vi "TextDiff.vi"(8 "error in (no error)":errorcluster, 9 "Output Folders":T5, 10 "VI 2 Screenshots in":T1, 11 "VI 1 Screenshots in":T1) -> (0 "error out":errorcluster, 2 "Description":string, 3 "appended path":path)   [LabVIEW 2020, in "VIDiffScreenshots.lvlib"]
uses:
  VIDiffScreenshots.lvlib
  Utilities/Output Folders.ctl
  VIScreenshots.ctl
  ScreenshotInfo.ctl
  Screenshot Type.ctl
  Utilities/FilePaths.ctl
  Utilities/VIDiffUtilities.lvlib
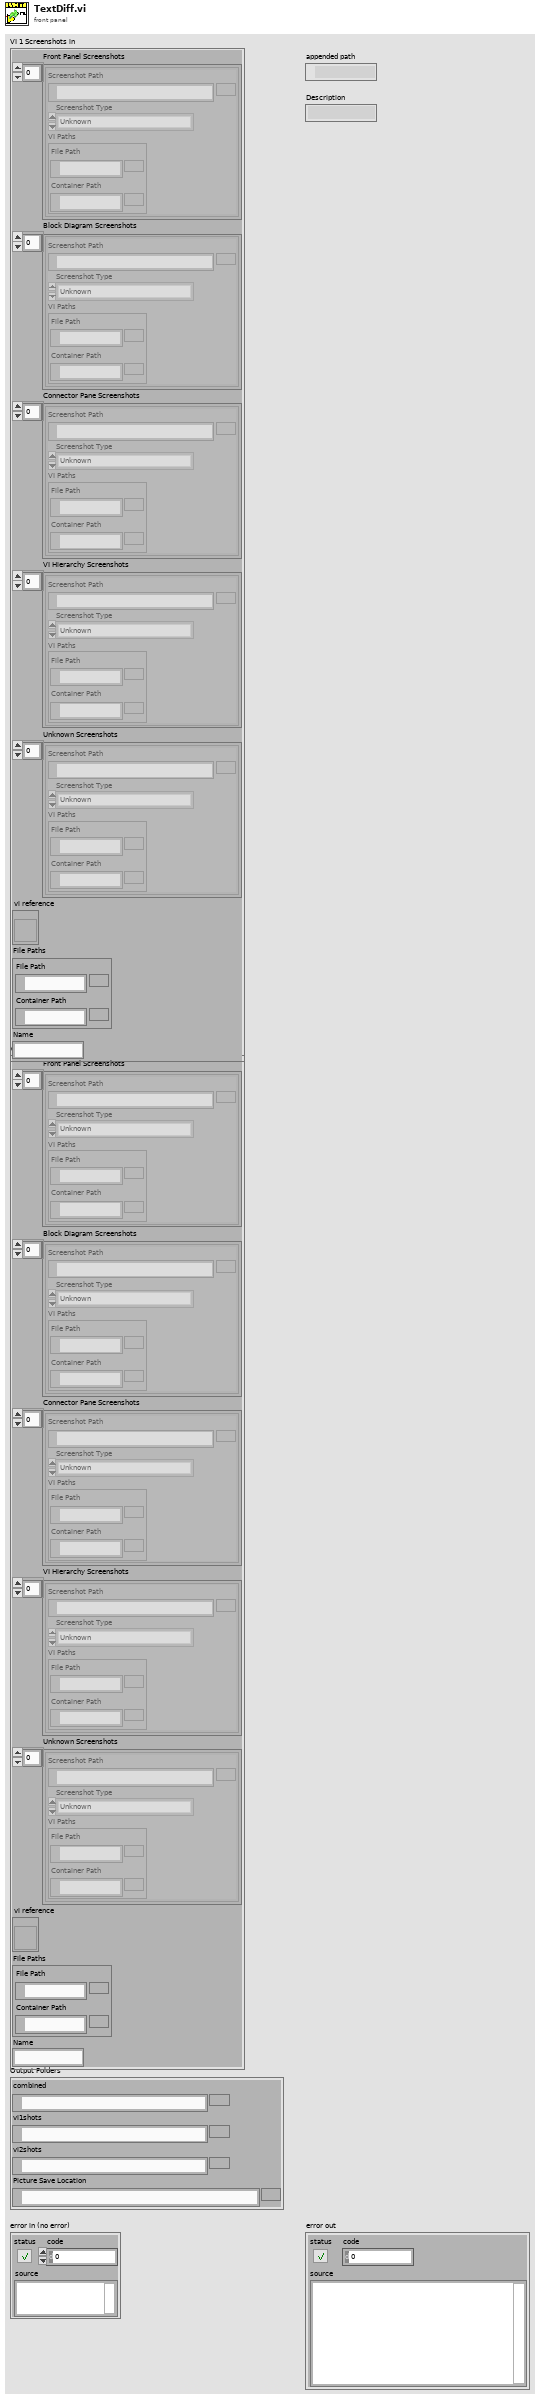
[diagram p1: front panel]
types:
  T1 = typedef "VIDiffScreenshots.lvlib/VIScreenshots.ctl" = cluster{"Front Panel Screenshots":T2[], "Block Diagram Screenshots":T2[], "Connector Pane Screenshots":T2[], "VI Hierarchy Screenshots":T2[], "Unknown Screenshots":T2[], "vi reference":refnum<vi>, "File Paths":cluster{"File Path":path, "Container Path":path}, "Name":string}
  T2 = typedef "VIDiffScreenshots.lvlib/ScreenshotInfo.ctl" = cluster{"Screenshot Path":path, "Screenshot Type":T3, "VI Paths":T4}
  T3 = typedef "VIDiffScreenshots.lvlib/Screenshot Type.ctl" = enum16{"Unknown", "Front Panel", "Connector Pane", "Block Diagram", "VI Hierarchy"}
  T4 = typedef "VIDiffUtilities.lvlib/FilePaths.ctl" = cluster{"File Path":path, "Container Path":path}
  T5 = typedef "VIDiffUtilities.lvlib/Output Folders.ctl" = cluster{"combined":path, "vi1shots":path, "vi2shots":path, "Picture Save Location":path}
  T6 = enum32{"invalid lock state", "Not Locked", "Locked (No Password)", "Password-protected"}
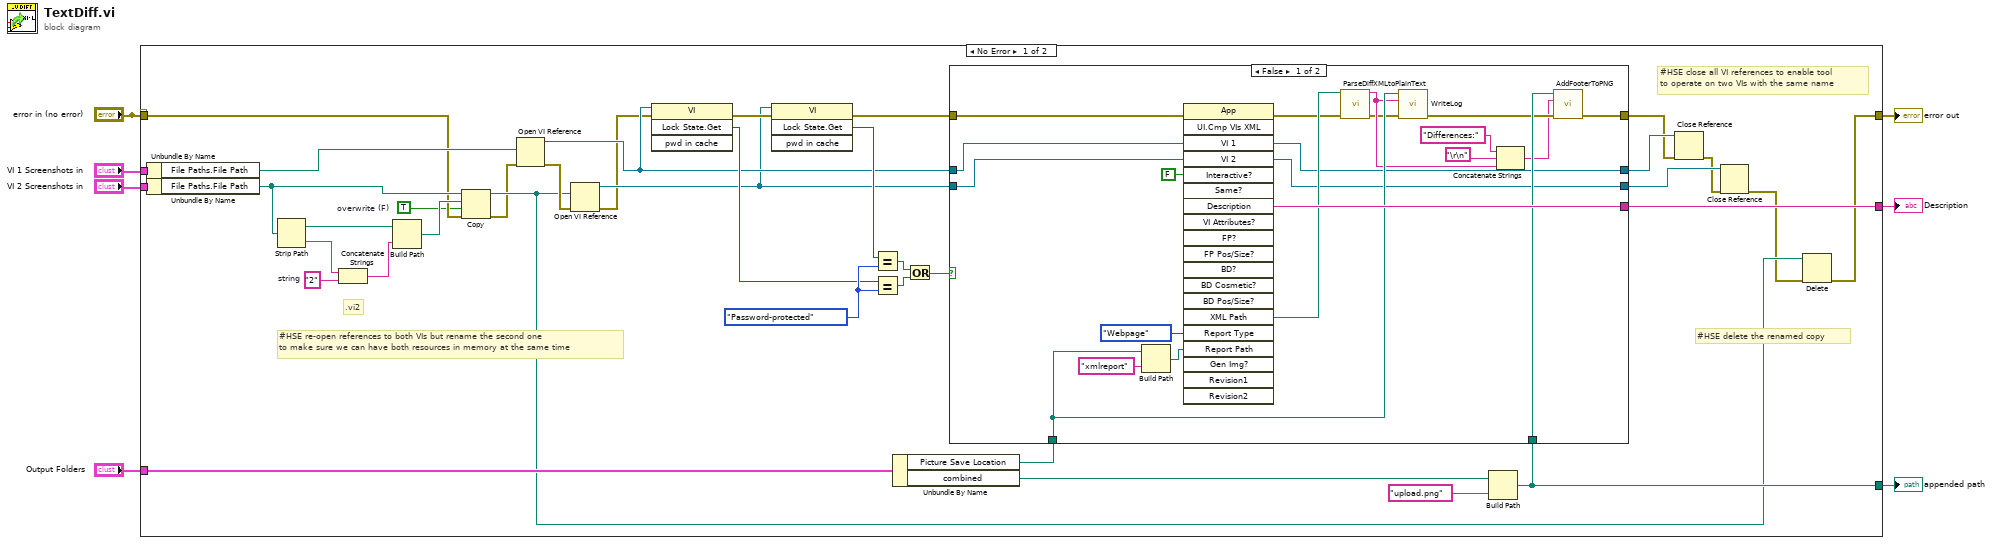
[diagram p0: block diagram]
diagram:
  n1 = case shown="No Error" "error in (no error)" {
    selector: "error in (no error)" -> [w10 w67]
    tunnel: "Output Folders" -> [w44 _]
    tunnel: "VI 2 Screenshots in" -> [w43 _]
    tunnel: "VI 1 Screenshots in" -> [w42 _]
    tunnel: "error in (no error)" -> [_ _]
    tunnel: [w41 _] -> w4
    tunnel: [w40 _] -> w3
    tunnel: [w11 w67] -> w2
    frame No Error {
      w8 = TRUE  # overwrite (F)
      w20 = "2"  # string
      w37 = T6."Password-protected" ("y")
      # "#HSE delete the renamed copy"
      # "#HSE close all VI references to enable tool \nto operate on two VIs with the same name"
      # "#HSE re-open references to both VIs but rename the second one \nto make sure we can have both resources in memory at the same time"
      # ".vi2"
      n2 = Unbundle By Name(w42) -> ("File Paths.File Path"=w28:path)
      n3 = Unbundle By Name(w43) -> ("File Paths.File Path"=w25:path)
      n4 = Strip Path(path=w25) -> (stripped path=w24:path, name=w22:string)
      n5 = Concatenate Strings(w22, w20) -> (w21:string)
      n6 = Build Path(base path=w24, name or relative path=w21) -> (appended path=w23:path)
      n7 = Copy(8:w10, 9:w8, 10:w23, 11:w25) -> (0:w9:errorcluster, 3:w15:path)  [unwired: 1 in, 1 out]
      n8 = Open VI Reference(vi path=w28, error in (no error)=w9) -> (vi reference=w27:refnum<vi>, error out=w19:errorcluster)  [unwired: 4 in]
      n9 = Open VI Reference(vi path=w15, error in (no error)=w19) -> (vi reference=w26:refnum<vi>, error out=w18:errorcluster)  [unwired: 4 in]
      n10 = invoke class="VI" method="Lock State.Get"(reference=w27, error in=w18) -> (error out=w38:errorcluster, "Get Lock State"=w33:T6)  [unwired: 2 in, 2 out]
      n11 = invoke class="VI" method="Lock State.Get"(reference=w26, error in=w38) -> (error out=w39:errorcluster, "Get Lock State"=w34:T6)  [unwired: 2 in, 2 out]
      n12 = Equal?(x=w34, y=w37) -> (x = y?=w35:bool)
      n13 = Equal?(x=w33, y=w37) -> (x = y?=w36:bool)
      n14 = Unbundle By Name(w44) -> ("Picture Save Location"=w31:path, "combined"=w32:path)
      n15 = Or(x=w35, y=w36) -> (x .or. y?=w29:bool)
      n16 = Build Path(base path=w32, name or relative path="upload.png") -> (appended path=w40:path)
      n17 = case shown="False" w29 {
        tunnel: [w63 _] -> w41
        tunnel: w40 -> [w62 _]
        tunnel: [w61 w66] -> w12
        tunnel: w39 -> [w60 w66]
        tunnel: w31 -> [w59 _]
        tunnel: w27 -> [w46 w65]
        tunnel: w26 -> [w45 w64]
        tunnel: [w46 w65] -> w17
        tunnel: [w45 w64] -> w16
        frame False {
          n18 = Build Path(base path=w59, name or relative path="xmlreport") -> (appended path=w57:path)
          n19 = invoke class="App" method="UI.Cmp VIs XML"(error in=w60, "VI 1"=w46, "VI 2"=w45, "Interactive?"=FALSE, "Report Type"=enum32{"None", "Webpage", "Text", "MS Word"}."Webpage", "Report Path"=w57) -> (error out=w50:errorcluster, "Description"=w63:string, "XML Path"=w58:path)  [unwired: 14 in, 17 out]
          n20 = call "ParseDiffXMLtoPlainText.vi"("XML Path"=w58, "error in"=w50) -> ("change description"=w53:string, "error out"=w51:errorcluster)  [unwired: 12 in]
          n21 = call "WriteLog.vi"("error in (no error)"=w51, "Log"=w53, "Log Folder"=w59) -> ("error out"=w52:errorcluster)  [unwired: 8 in]
          n22 = Concatenate Strings("Differences:" ("string"), "\r\n", w53) -> (w48:string)
          n23 = call "AddFooterToPNG.vi"("error in (no error)"=w52, "Footer String"=w48, "PNG File"=w62) -> ("error out"=w61:errorcluster)  [unwired: 8 in]
        }
        frame True {
          # "Can't get the XML for locked VIs"
        }
      }
      n24 = Close Reference(reference=w17, error in (no error)=w12) -> (error out=w14:errorcluster)
      n25 = Close Reference(reference=w16, error in (no error)=w14) -> (error out=w13:errorcluster)
      n26 = Delete(path (use dialog)=w15, error in=w13) -> (error out=w11:errorcluster)  [unwired: 3 in, 2 out]
    }
    frame Error {
    }
  }
  "Description" <- w4
  "appended path" <- w3
  "error out" <- w2
